vi "ALapp_PID.vi"(0 "?":T1={"P Gain"=0.1, "I Gain"=0.001, "D Gain"=0.0}, 1 "Setpoint":dbl, 2 "Feedback":dbl, 3 "integral reset":bool, 4 "PID Out Max":dbl=1.0, 6 "Integrator Range":dbl=0.5) -> (7 "Motor Output":dbl)   [LabVIEW 2011]
panel:
  out "P Term":dbl(knob) scale=-1.0..1.0
  out "I Term":dbl(knob) scale=-1.0..1.0
  out "D Term":dbl(knob) scale=-1.0..1.0
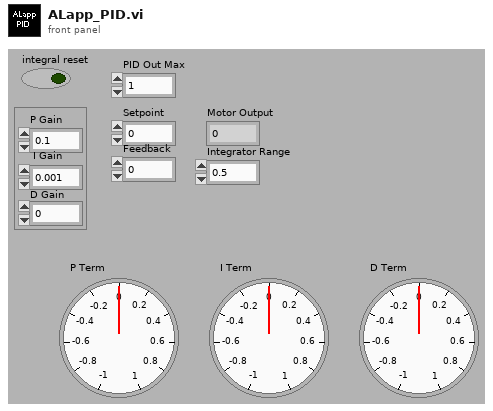
[diagram p1: front panel]
types:
  T1 = cluster{"P Gain":dbl, "I Gain":dbl, "D Gain":dbl}
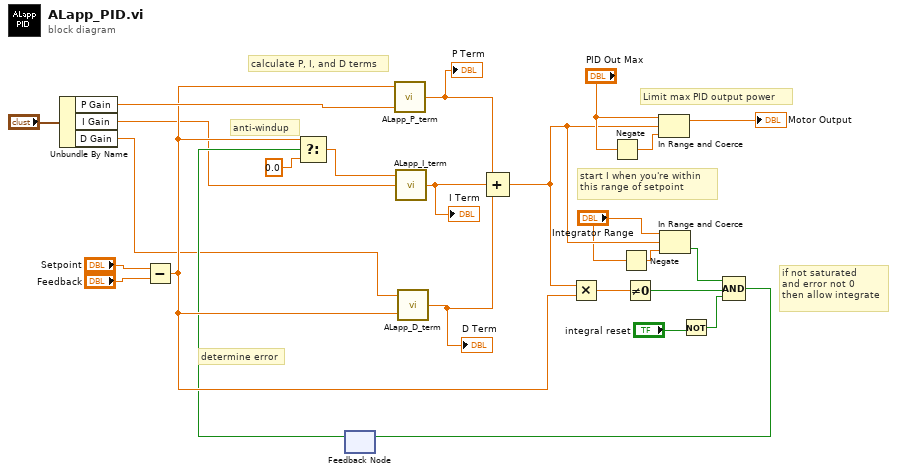
[diagram p0: block diagram]
diagram:
  # "start I when you're within \nthis range of setpoint"
  # "anti-windup"
  # "if not saturated\nand error not 0\nthen allow integrate"
  # "Limit max PID output power"
  # "calculate P, I, and D terms"
  # "determine error"
  n1 = Unbundle By Name("?") -> ("P Gain"=w17:dbl, "I Gain"=w9:dbl, "D Gain"=w8:dbl)
  n2 = Subtract(x="Setpoint", y="Feedback") -> (x-y=w15:dbl)
  n3 = feedback #1() -> (w13:bool)  [unwired: 1 out]
  n4 = Select(t=w15, s=w13, f=0.0) -> (s? t:f=w19:dbl)
  n5 = call "ALapp_P_term.vi"("P Term Gain"=w17, "Error"=w15) -> ("P Term"=w1:dbl)  [unwired: 1 out]
  "P Term" <- w1
  n6 = call "ALapp_I_term.vi"("I Term Gain"=w9, "error"=w19) -> ("I Term Output"=w20:dbl)  [unwired: 1 out]
  "I Term" <- w20
  n7 = call "ALapp_D_term.vi"("Error"=w15, "D Term Gain"=w8) -> ("D Term"=w21:dbl)
  "D Term" <- w21
  n8 = Compound Arithmetic op=ADD(w1, w20, w21) -> (w4:dbl)
  n9 = Multiply(x=w4, y=w15) -> (x*y=w12:dbl)
  n10 = Negate(x="PID Out Max") -> (-x=w23:dbl)
  n11 = Negate(x="Integrator Range") -> (-x=w2:dbl)
  n12 = Not Equal To 0?(x=w12) -> (x != 0?=w11:bool)
  n13 = In Range and Coerce(upper limit="PID Out Max", x=w4, lower limit=w23) -> (coerced(x)=→"Motor Output":dbl)  [unwired: 1 out]
  n14 = In Range and Coerce(upper limit="Integrator Range", x=w4, lower limit=w2) -> (In Range?=w5:bool)  [unwired: 1 out]
  n15 = Not(x="integral reset") -> (.not. x?=w6:bool)
  n16 = Compound Arithmetic op=AND(w5, w11, w6) -> (w14:bool)
  n17 = feedback-in #1(w14) -> ()
